vi "Histogram0002.vi"   [LabVIEW 2013]
uses:
  <vilib>/Heliosphere Research LLC/Advanced Plotting Toolkit/api_plotting/Histogram_Automatic.vi
  <vilib>/Heliosphere Research LLC/Advanced Plotting Toolkit/Advanced Plotting Toolkit.lvlib
types:
  T1 = typedef "Advanced Plotting Toolkit.lvlib/PlotID.ctl" = i32
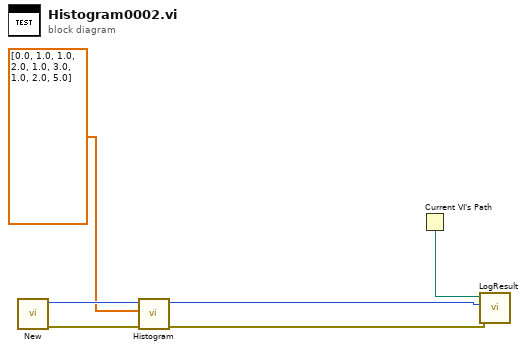
[diagram p0: block diagram]
diagram:
  n1 = call <vilib>:"New.vi"() -> ("error out"=w3:errorcluster, "Plot ID"=w6:T1)  [unwired: 10 in]
  n2 = call-poly <vilib>:"Histogram.vi"("error in (no error)"=w3, "Data"=dbl[] [0.0, 1.0, 1.0, 2.0, 1.0, 3.0, 1.0, 2.0, 5.0], "Plot ID"=w6) -> ("error out"=w2:errorcluster, "Plot ID Out"=w5:T1)  [unwired: 7 in]
  n3 = Current VI's Path() -> (path=w4:path)
  n4 = call "LogResult.vi"("Test Result"=w2, "Test Artifact"=w5, "VI Path"=w4) -> ()  [unwired: 9 in]
